vi "SR785 Init.vi"(0 "VISA resource name":refnum<visa-resource-name>, 1 "Center (51.2E+3 Hz)":dbl=51200.0 format="%^.2e", 2 "Span (102.4E+3 Hz)":dbl=102400.0 format="%^.2e", 3 "Resolution (2: 400)":i32(ring)=2 items=["100", "200", "400", "800"], 11 "error in (no error)":errorcluster) -> (15 "error out":errorcluster)   [LabVIEW 2023]
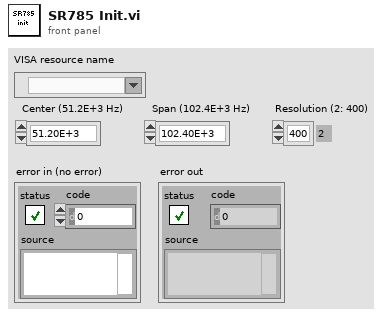
[diagram p1: front panel]
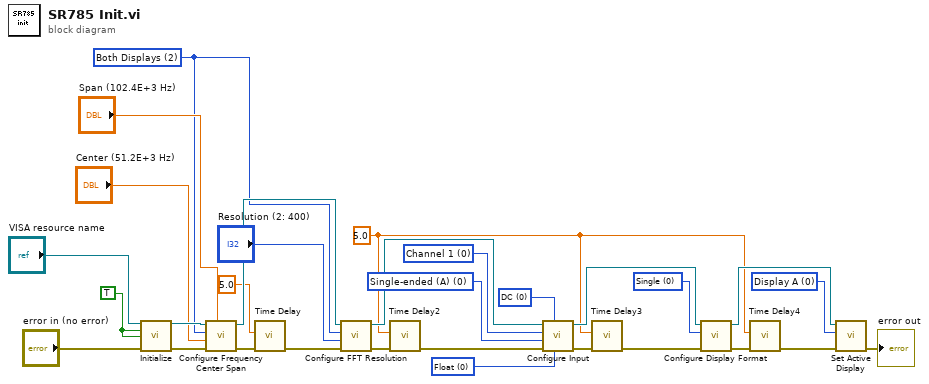
[diagram p0: block diagram]
diagram:
  w1 = 5.0 ("Delay Time (s)")
  w7 = 0 items=["Float", "Ground"] ("Input Ground (0: Float)")
  w8 = 0 items=["Single-ended (A)", "Differential (A - B)"] ("Input Mode (0: Single-ended (A))")
  w9 = 0 items=["Channel 1", "Channel 2", "Both Channel"] ("Channel (0: Channel 1)")
  w10 = 0 items=["DC", "AC", "ICP"] ("Coupling (0: DC)")
  w15 = 0 items=["Display A", "Display B"] ("Active Display (0: Display A)")
  w17 = 2 items=["Display A", "Display B", "Both Displays"] ("Display")
  w27 = 0 items=["Single", "Dual", "Overlay"] ("Format (1: Dual)")
  w29 = TRUE ("ID Query (T: Check)")
  n1 = call <instrlib>:"Initialize.vi"("VISA resource name"="VISA resource name", "ID Query (T: Check)"=w29, "Reset (T: Reset)"=w29, "error in (no error)"="error in (no error)") -> ("VISA resource name out"=w23:refnum<visa-resource-name>, "error out"=w21:errorcluster)  [unwired: 10 in]
  n2 = call <instrlib>:"Configure Frequency Center Span.vi"("Span (102.4E+3 Hz)"="Span (102.4E+3 Hz)", "error in (no error)"=w21, "Center (51.2E+3 Hz)"="Center (51.2E+3 Hz)", "Display (2: Both Displays)"=w17, "VISA resource name"=w23) -> ("error out"=w20:errorcluster, "VISA resource name out"=w22:refnum<visa-resource-name>)  [unwired: 5 in]
  n3 = call "Time Delay"("error in (no error)"=w20, "Delay Time (s)"=5.0) -> ("error out"=w6:errorcluster)  [unwired: 9 in]
  n4 = call <instrlib>:"Configure FFT Resolution.vi"("error in (no error)"=w6, "Resolution (2: 400)"="Resolution (2: 400)", "Display (2: Both Displays)"=w17, "VISA resource name"=w22) -> ("error out"=w14:errorcluster, "VISA resource name out"=w12:refnum<visa-resource-name>)  [unwired: 6 in]
  n5 = call "Time Delay2"("error in (no error)"=w14, "Delay Time (s)"=w1) -> ("error out"=w4:errorcluster)  [unwired: 9 in]
  n6 = call <instrlib>:"Configure Input.vi"("Input Ground (0: Float)"=w7, "Coupling (0: DC)"=w10, "error in (no error)"=w4, "Input Mode (0: Single-ended (A))"=w8, "Channel (0: Channel 1)"=w9, "VISA resource name"=w12) -> ("error out"=w13:errorcluster, "VISA resource name out"=w11:refnum<visa-resource-name>)  [unwired: 4 in]
  n7 = call "Time Delay3"("error in (no error)"=w13, "Delay Time (s)"=w1) -> ("error out"=w3:errorcluster)  [unwired: 9 in]
  n8 = call <instrlib>:"Configure Display Format.vi"("error in (no error)"=w3, "Format (1: Dual)"=w27, "VISA resource name"=w11) -> ("error out"=w25:errorcluster, "VISA resource name out"=w26:refnum<visa-resource-name>)  [unwired: 7 in]
  n9 = call "Time Delay4"("error in (no error)"=w25, "Delay Time (s)"=w1) -> ("error out"=w2:errorcluster)  [unwired: 9 in]
  n10 = call <instrlib>:"Set Active Display.vi"("error in (no error)"=w2, "Active Display (0: Display A)"=w15, "VISA resource name"=w26) -> ("error out"=→"error out":errorcluster)  [unwired: 7 in, 1 out]
